vi "Convert To JSON Comp Format.vi"(11 "output settings":T2={"output rate"=51200.0, "range"=5.0, "terminal configuration"=enum."Pseudodifferential", "output impedance"=0.0, "common mode offset"=0.0, "pure tone mode"=FALSE}) -> (3 "output settings JSON":T1={"output rate"=51200.0, "range"=5.0, "terminal configuration"="", "output impedance"=0.0, "common mode offset"=0.0, "pure tone mode"=FALSE})   [LabVIEW 2022 SP3, in "Analog Gen Settings.lvlib"]
uses:
  Analog Gen Settings.lvlib
  service/generation/controls/analog output settings.ctl
  service/generation/controls/terminal configuration.ctl
  analog output settings_json.ctl
  service/generation/controls/AudioGenTypeDefs.lvlib
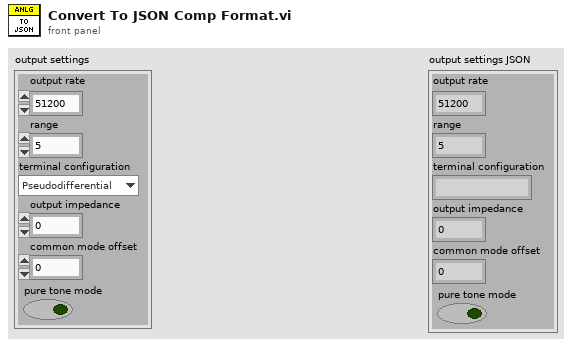
[diagram p1: front panel]
types:
  T1 = typedef "Analog Gen Settings.lvlib/analog output settings_json.ctl" = cluster{"output rate":dbl, "range":dbl, "terminal configuration":string, "output impedance":dbl, "common mode offset":dbl, "pure tone mode":bool}
  T2 = typedef "AudioGenTypeDefs.lvlib/analog output settings.ctl" = cluster{"output rate":dbl, "range":dbl, "terminal configuration":T3, "output impedance":dbl, "common mode offset":dbl, "pure tone mode":bool}
  T3 = typedef "AudioGenTypeDefs.lvlib/terminal configuration.ctl" = enum32{"Default", "RSE", "Differential", "Pseudodifferential"}
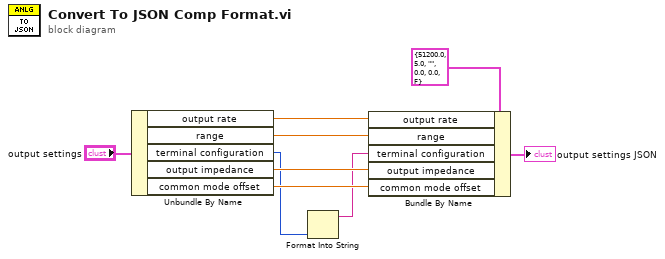
[diagram p0: block diagram]
diagram:
  n1 = Unbundle By Name("output settings") -> ("output rate"=w8:dbl, "range"=w7:dbl, "terminal configuration"=w4:T3, "output impedance"=w6:dbl, "common mode offset"=w5:dbl)
  n2 = Format Into String(w4) -> (resulting string=w3:string)  [unwired: 3 in, 1 out]
  n3 = Bundle By Name(cluster=T1 {"output rate"=51200.0, "range"=5.0, "terminal configuration"="", "output impedance"=0.0, "common mode offset"=0.0, "pure tone mode"=FALSE} ("output settings JSON"), "output rate"=w8, "range"=w7, "terminal configuration"=w3, "output impedance"=w6, "common mode offset"=w5) -> (→"output settings JSON":T1)
